vi "Valid.vi"(11 "Gesture Wrapper in":refnum<class "Gesture Wrapper.lvclass">) -> (2 "valid?":bool, 3 "Gesture Wrapper out":refnum<class "Gesture Wrapper.lvclass">)   [LabVIEW 2023, in "Gesture Wrapper.lvclass"]
doc: "Check validity of contained gesture."
uses:
  Gesture Wrapper.lvclass
  Gesture Wrapper.lvclass/Gesture Wrapper.ctl
  Gesture/Gesture.lvclass
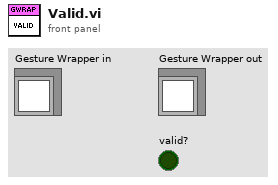
[diagram p1: front panel]
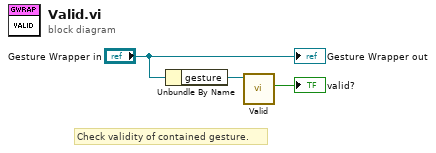
[diagram p0: block diagram]
diagram:
  # "Check validity of contained gesture."
  n1 = Unbundle By Name("Gesture Wrapper in") -> ("gesture"=w2:refnum<class "Gesture.lvclass">)
  n2 = call-dynamic "Valid.vi"("gesture in"=w2) -> ("valid"=→"valid?":bool)  [unwired: 10 in]
  "Gesture Wrapper out" <- "Gesture Wrapper in"
